vi "Read DVR.vi"(8 "error in (no error)":errorcluster, 11 "Subject in":refnum<class "Subject.lvclass">) -> (0 "error out":errorcluster, 2 "DVR":refnum<data-value>, 3 "Subject out":refnum<class "Subject.lvclass">)   [LabVIEW 2012]
uses:
  Subject.lvclass
  Observer/Observer.lvclass
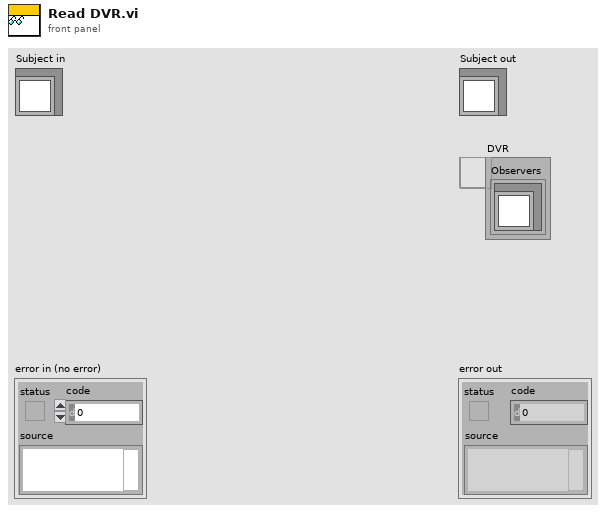
[diagram p1: front panel]
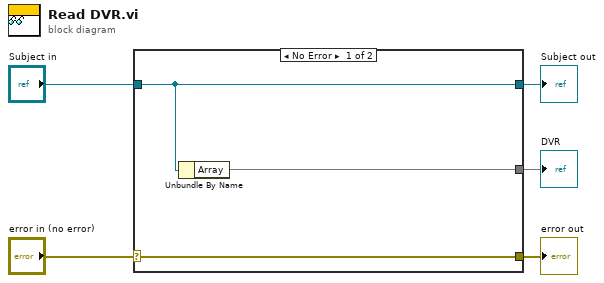
[diagram p0: block diagram]
diagram:
  n1 = case shown="No Error" "error in (no error)" {
    selector: "error in (no error)" -> [w8 w9]
    tunnel: [w8 w9] -> w4
    tunnel: [w7 w10] -> w2
    tunnel: "Subject in" -> [w7 w10]
    tunnel: [w6 _] -> w1
    frame No Error {
      n2 = Unbundle By Name(w7) -> ("Array"=w6)
    }
    frame Error {
    }
  }
  "error out" <- w4
  "Subject out" <- w2
  "DVR" <- w1
